vi "Clear Report.vi"(0 "report in":refnum<class "NI_HTML.lvclass">, 11 "error in (no error)":errorcluster) -> (4 "report out":refnum<class "NI_HTML.lvclass">, 15 "error out":errorcluster)   [LabVIEW 2020, in "NI_HTML.lvclass"]
doc: "Clears the report of all text, headers, footers, and formatting information."
uses:
  NI_HTML.lvclass
  HTML Report Data.ctl
  NI_HTML.lvclass/NI_HTML.ctl
  NI_ReportGenerationCore.lvlib
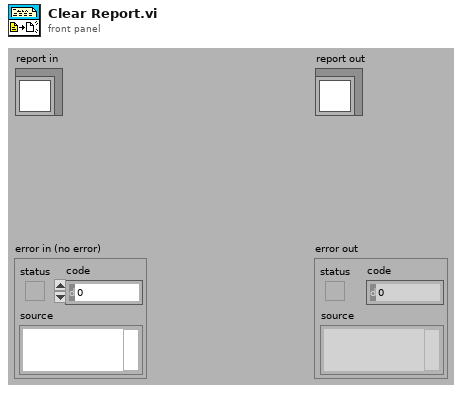
[diagram p1: front panel]
types:
  T1 = typedef "NI_ReportGenerationCore.lvlib/HTML Report Data.ctl" = cluster{"Body Text":string, "Font Tag":string, "Title Text":string, "Header Text":string, "Footer Text":string, "Image List":path[]}
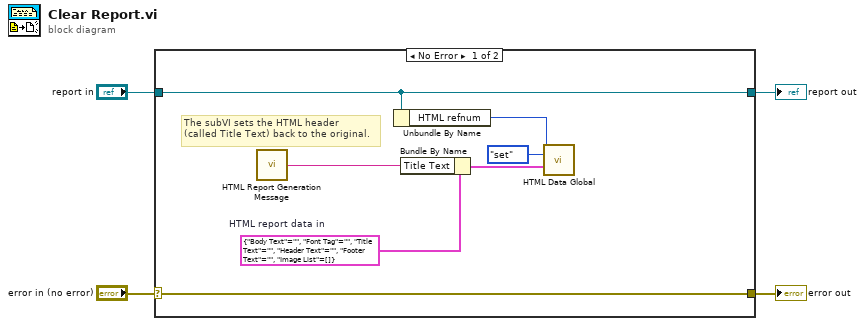
[diagram p0: block diagram]
diagram:
  n1 = case shown="No Error" "error in (no error)" {
    selector: "error in (no error)" -> [w11 w13]
    tunnel: [w11 w13] -> w3
    tunnel: [w9 w12] -> w1
    tunnel: "report in" -> [w9 w12]
    frame No Error {
      w8 = T1 {"Body Text"="", "Font Tag"="", "Title Text"="", "Header Text"="", "Footer Text"="", "Image List"=[]}  # HTML report data in
      # "The subVI sets the HTML header \n(called Title Text) back to the original."
      n2 = call "HTML Report Generation Message.vi"() -> ("String"=w7:string)
      n3 = Unbundle By Name(w9) -> ("HTML refnum"=w5:u32)
      n4 = Bundle By Name(cluster=w8, "Title Text"=w7) -> (w6:T1)
      n5 = call "HTML Data Global.vi"("HTML refnum"=w5, "menu"=enum16{"init", "get", "set", "delete"}."set", "HTML report data in"=w6) -> ()  [unwired: 13 out]
    }
    frame Error {
    }
  }
  "error out" <- w3
  "report out" <- w1
